vi "Set Attributes.vi"(8 "error in (no error)":errorcluster, 11 "ITest Executive Builder Dialog in":refnum<class "ITest Executive Builder Dialog.lvclass">) -> (0 "error out":errorcluster, 3 "ITest Executive Builder Dialog out":refnum<class "ITest Executive Builder Dialog.lvclass">)   [LabVIEW 2017, in "ITest Executive Builder Dialog.lvclass"]
uses:
  <vilib>/gpm_packages/@cs/Test-executive-builder/Source/Test Executive Builder Dialogs/ITest Executive Builder Dialog/ITest Executive Builder Dialog.lvclass
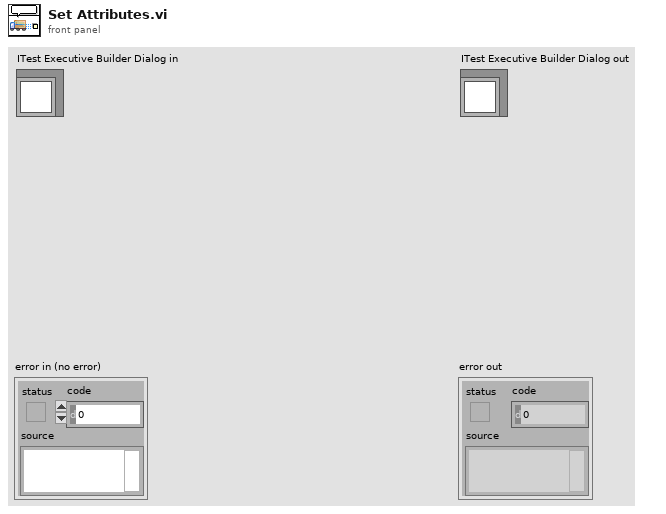
[diagram p1: front panel]
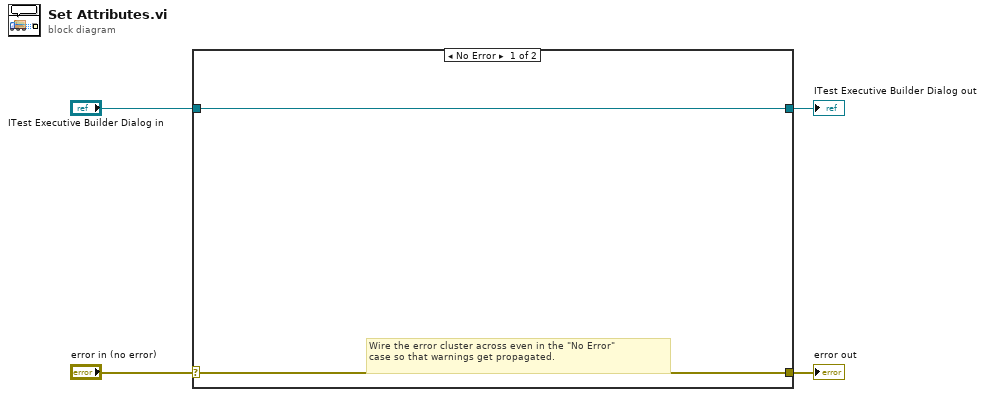
[diagram p0: block diagram]
diagram:
  n1 = case shown="No Error" "error in (no error)" {
    selector: "error in (no error)" -> [w5 w8]
    tunnel: [w5 w8] -> w3
    tunnel: [w6 w7] -> w1
    tunnel: "ITest Executive Builder Dialog in" -> [w6 w7]
    frame No Error {
      # "Wire the error cluster across even in the \"No Error\"\ncase so that warnings get propagated."
    }
    frame Error {
    }
  }
  "error out" <- w3
  "ITest Executive Builder Dialog out" <- w1
